vi "GetGalvoLocIRdata.vi"(10 "Galvo location":i32, 11 "irData":i32[](array[numeric])) -> (1 "temperature":i32, 2 "yLoc":i32, 3 "xLoc":i32)   [LabVIEW 2020]
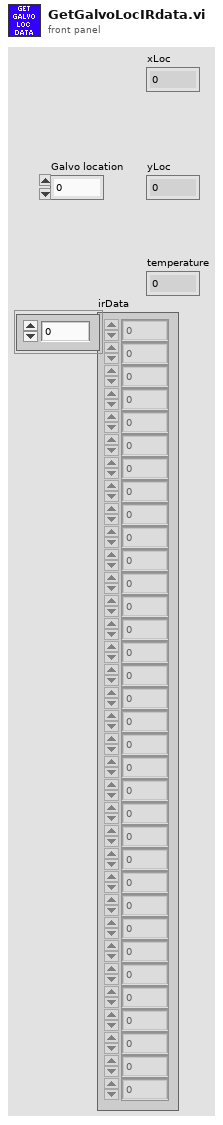
[diagram p1: front panel]
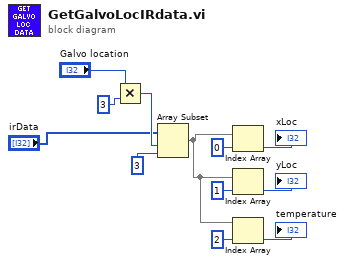
[diagram p0: block diagram]
diagram:
  n1 = Multiply(x="Galvo location", y=3) -> (x*y=w11:i32)
  n2 = Array Subset(array="irData", index=w11, length=3) -> (w9:i32[])
  n3 = Index Array(array=w9, index=0) -> (element=→"xLoc":i32)
  n4 = Index Array(array=w9, index=1) -> (element=→"yLoc":i32)
  n5 = Index Array(array=w9, index=2) -> (element=→"temperature":i32)
